vi "cc1.vi"() -> ()   [LabVIEW 2020]
uses:
  LabVIEW Example(8.6)/ControlCAN/ControlCAN.llb/VCI_CAN_OBJ.ctl
  LabVIEW Example(8.6)/ControlCAN/ControlCAN.llb/Return Val.ctl
  LabVIEW Example(8.6)/ControlCAN/ControlCAN.llb/DevType.ctl
  TEST1/ControlCAN/ControlCAN.llb/VCI_INIT_CONFIG.ctl
  TEST1/ControlCAN/ControlCAN.llb/InitFlag.ctl
  TEST1/ControlCAN/ControlCAN.llb/Fliter.ctl
  TEST1/ControlCAN/ControlCAN.llb/Mode.ctl
  LabVIEW Example(8.6)/ControlCAN/ControlCAN.lvlib
panel:
  out "Return Val 2":T1=1 items=["OK"=1, "ERROR1"=0, "ERROR2"=-1]
  out "Recieve[0].Data":u8[](array[numeric])
  out "Recieve":T2[](array[typedef])
  in  "Len":u32=2500 caption="Len(2500)"
  out "Recieve 2":T2[](array[typedef])
  out "子字符串":string
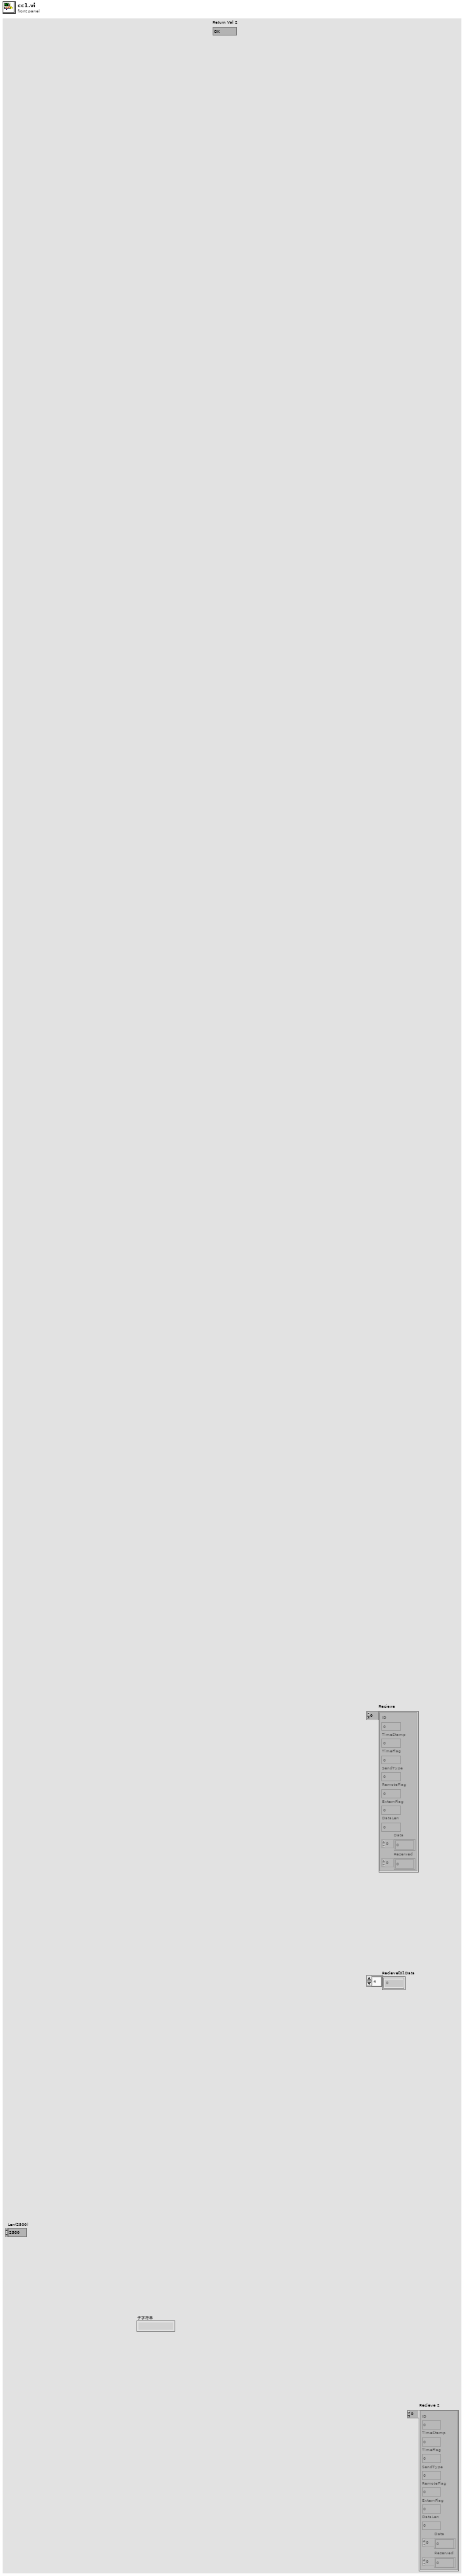
[diagram p1: front panel]
types:
  T1 = typedef "ControlCAN.lvlib/Return Val.ctl" = i32
  T2 = typedef "ControlCAN.lvlib/VCI_CAN_OBJ.ctl" = cluster{"ID":u32, "TimeStamp":u32, "TimeFlag":u8, "SendType":u8, "RemoteFlag":u8, "ExternFlag":u8, "DataLen":u8, "Data":u8[], "Reserved":u8[]}
  T3 = typedef "ControlCAN.lvlib/VCI_INIT_CONFIG.ctl" = cluster{"AccCode":u32, "AccMask":u32, "InitFlag":T4, "Fliter":T5, "Timing0":u8, "Timing1":u8, "Mode":T6}
  T4 = typedef "ControlCAN.lvlib/InitFlag.ctl" = u32
  T5 = typedef "ControlCAN.lvlib/Fliter.ctl" = u8
  T6 = typedef "ControlCAN.lvlib/Mode.ctl" = u8
  T7 = typedef "ControlCAN.lvlib/DevType.ctl" = u32
  T8 = cluster{"Recieve[0]":T2, "Recieve[1]":T2, "Recieve[2]":T2, "Recieve[3]":T2, "Recieve[4]":T2, "Recieve[5]":T2, "Recieve[6]":T2, "Recieve[7]":T2, "Recieve[8]":T2}
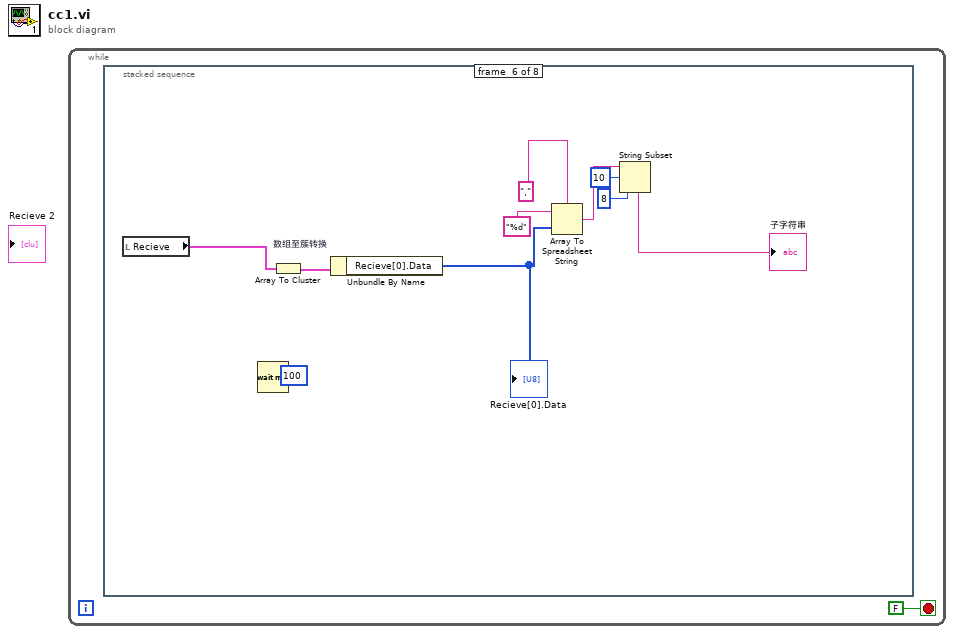
[diagram p0: block diagram]
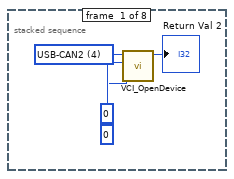
[diagram p2: hidden frame]
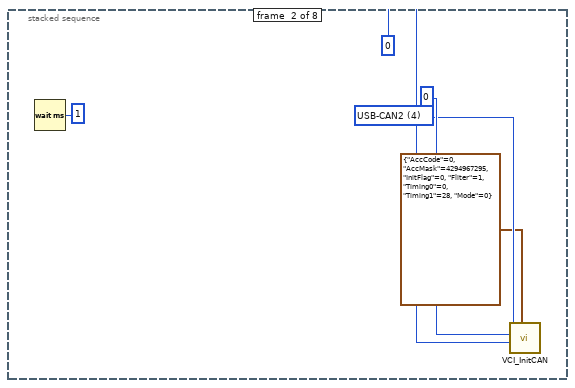
[diagram p3: hidden frame]
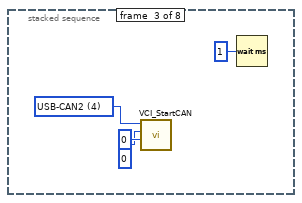
[diagram p4: hidden frame]
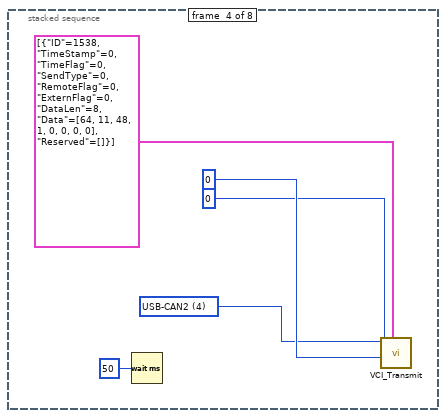
[diagram p5: hidden frame]
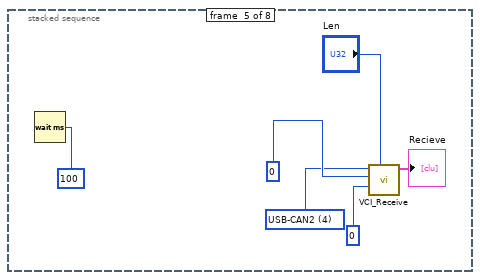
[diagram p6: hidden frame]
diagram:
  n1 = while {
    stop <- FALSE stop-if-true
    n2 = stacked-sequence {
      frame #0 {
        w2 = T7 4 items=["USB-CAN"=3, "USB-CAN2"=4] ("DevType")
        n3 = call "VCI_OpenDevice.vi"("Reserved"=u32 0, "DevIndex"=u32 0, "DevType"=w2) -> ("Return Val"=→"Return Val 2":T1)  [unwired: 7 in, 1 out]
      }
      frame #1 {
        w8 = T7 4 items=["USB-CAN"=3, "USB-CAN2"=4] ("DevType")
        n4 = Wait (ms)(milliseconds to wait=u32 1 ("等待时间（毫秒）")) -> ()  [unwired: 1 out]
        n5 = call "VCI_InitCAN.vi"("VCI_INIT_CONFIG"=T3 {"AccCode"=0, "AccMask"=4294967295, "InitFlag"=0, "Fliter"=1, "Timing0"=0, "Timing1"=28, "Mode"=0}, "CANIndex"=u32 0, "DevIndex"=u32 0, "DevType"=w8) -> ()  [unwired: 6 in, 2 out]
      }
      frame #2 {
        w12 = T7 4 items=["USB-CAN"=3, "USB-CAN2"=4] ("DevType")
        n6 = call "VCI_StartCAN.vi"("CANIndex"=u32 0, "DevIndex"=u32 0, "DevType"=w12) -> ()  [unwired: 7 in, 2 out]
        n7 = Wait (ms)(milliseconds to wait=u32 1 ("等待时间（毫秒）")) -> ()  [unwired: 1 out]
      }
      frame #3 {
        w16 = T7 4 items=["USB-CAN"=3, "USB-CAN2"=4] ("DevType")
        n8 = Wait (ms)(milliseconds to wait=u32 50 ("等待时间（毫秒）")) -> ()  [unwired: 1 out]
        n9 = call "VCI_Transmit.vi"("Buffer"=T2[] [{"ID"=1538, "TimeStamp"=0, "TimeFlag"=0, "SendType"=0, "RemoteFlag"=0, "ExternFlag"=0, "DataLen"=8, "Data"=[64, 11, 48, 1, 0, 0, 0, 0], "Reserved"=[]}], "CANIndex"=u32 0, "DevIndex"=u32 0, "DevType"=w16) -> ()  [unwired: 6 in, 2 out]
      }
      frame #4 {
        w20 = T7 4 items=["USB-CAN"=3, "USB-CAN2"=4] ("DevType")
        n10 = Wait (ms)(milliseconds to wait=u32 100 ("等待时间（毫秒）")) -> ()  [unwired: 1 out]
        n11 = call "VCI_Receive.vi"("Len"="Len", "CANIndex"=u32 0, "DevIndex"=u32 0, "DevType"=w20) -> ("Recieve"=→"Recieve":T2[])  [unwired: 6 in, 1 out]
      }
      frame #5 {
        n12 = local read "Recieve"() -> (w35:T2[])
        n13 = Wait (ms)(milliseconds to wait=u32 100 ("等待时间（毫秒）")) -> ()  [unwired: 1 out]
        n14 = Array To Cluster "数组至簇转换"(array=w35) -> (cluster=w28:T8)
        n15 = Unbundle By Name(w28) -> ("Recieve[0].Data"=w30:u8[])
        "Recieve[0].Data" <- w30
        n16 = Array To Spreadsheet String(delimiter (Tab)="," ("分隔符(Tab)"), array=w30, 3:"%d" ("格式字符串")) -> (spreadsheet string=w32:string)
        n17 = String Subset(string=w32, offset (0)=10 ("偏移量(0)"), length (rest)=8 ("长度（剩余）")) -> (substring=→"子字符串":string)
      }
      frame #6 {
      }
      frame #7 {
      }
    }
  }
